vi "CAlex2_InitCuff.vi"(4 "ShankExtraWeight":dbl, 6 "ThighExtraWeight":dbl, 8 "error in (no error)":errorcluster, 10 "LegProperty":T1={"BodyDim(m)"={"ThighLt"=0.4, "ShankLt"=0.41, "HipWd"=0.32}, "BodyWt(kg)"={"Thigh"=0.0, "Shank"=0.0}, "CuffLoc(m)"={"HipCuffWd"=0.4, "HipCuffHt"=0.1, "HipCuffFwdShift"=0.0, "ThighCuffToKnee"=0.25, "ThighCuffDist"=0.0, "ShankCuffToKnee"=0.15}}, 11 "CAlex2 in":refnum<class "CAlex2.lvclass">) -> (0 "error out":errorcluster, 3 "CAlex2 out":refnum<class "CAlex2.lvclass">)   [LabVIEW 2015, in "CAlex2.lvclass"]
uses:
  CAlex2.lvclass
  TypeDef/LowerBodyDim.ctl
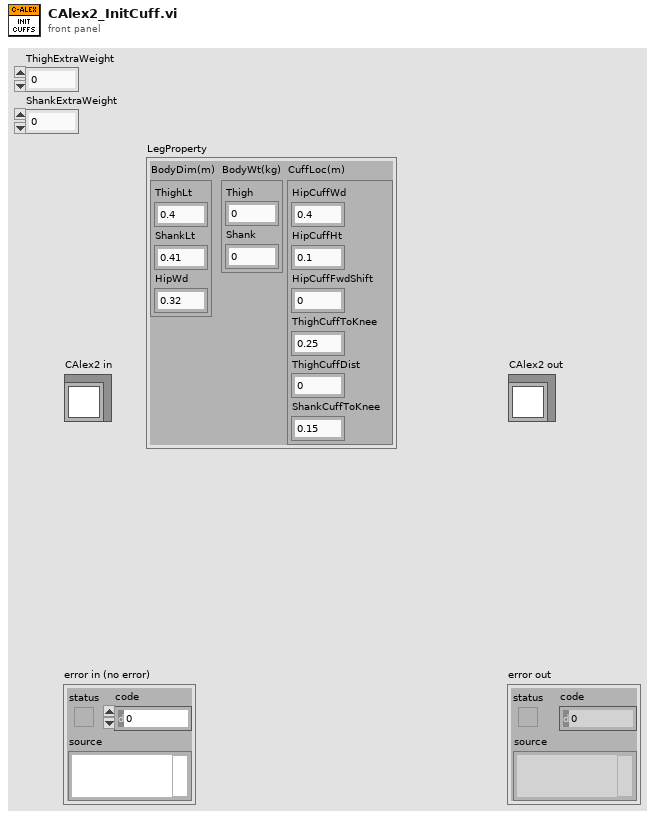
[diagram p1: front panel]
types:
  T1 = typedef "CAlex2.lvclass/LowerBodyDim.ctl" = cluster{"BodyDim(m)":cluster{"ThighLt":dbl, "ShankLt":dbl, "HipWd":dbl}, "BodyWt(kg)":cluster{"Thigh":dbl, "Shank":dbl}, "CuffLoc(m)":cluster{"HipCuffWd":dbl, "HipCuffHt":dbl, "HipCuffFwdShift":dbl, "ThighCuffToKnee":dbl, "ThighCuffDist":dbl, "ShankCuffToKnee":dbl}}
  T2 = enum16{"Thigh Cuff Low Lower Edge", "Thigh Cuff High Center"}
  T3 = typedef "CableSerialChain.lvclass/Cuff.ctl" = cluster{"BodyID":i32, "CoM(CuffCS)":T4, "Mass(kg)":dbl, "CablePts(CuffCS)":T4[], "Cuff->Body":T5}
  T4 = typedef "Bodies.lvclass/PointOnBody.ctl" = cluster{"Coord4":dbl[], "ID":i32}
  T5 = typedef "NI_Matrix.lvlib/RealMatrix.ctl" = dbl[][]
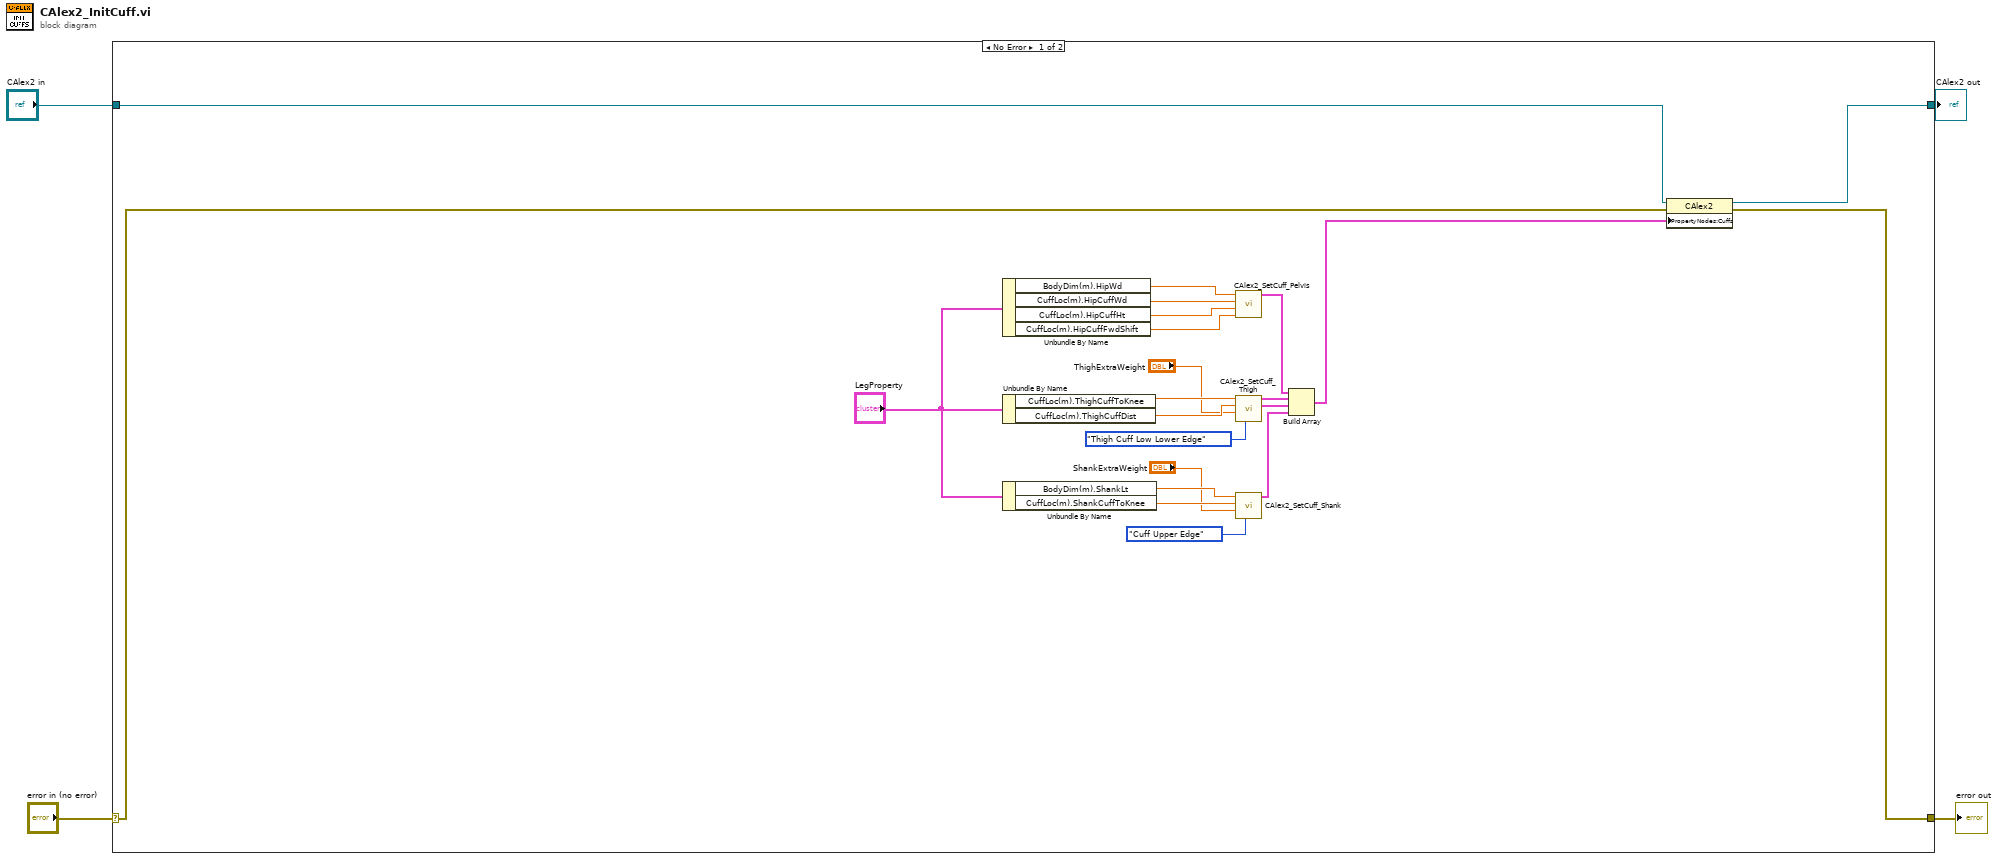
[diagram p0: block diagram]
diagram:
  n1 = case shown="No Error" "error in (no error)" {
    selector: "error in (no error)" -> [w7 w28]
    tunnel: [w24 w28] -> w3
    tunnel: [w25 w27] -> w1
    tunnel: "CAlex2 in" -> [w8 w27]
    frame No Error {
      n2 = Unbundle By Name("LegProperty") -> ("BodyDim(m).HipWd"=w15:dbl, "CuffLoc(m).HipCuffWd"=w13:dbl, "CuffLoc(m).HipCuffHt"=w14:dbl, "CuffLoc(m).HipCuffFwdShift"=w12:dbl)
      n3 = Unbundle By Name("LegProperty") -> ("CuffLoc(m).ThighCuffToKnee"=w11:dbl, "CuffLoc(m).ThighCuffDist"=w10:dbl)
      n4 = Unbundle By Name("LegProperty") -> ("BodyDim(m).ShankLt"=w19:dbl, "CuffLoc(m).ShankCuffToKnee"=w18:dbl)
      n5 = call "CAlex2_SetCuff_Pelvis.vi"("Hip Cuff Forward Shift"=w12, "Hip Cuff Height"=w14, "Hip Cuff Width"=w13, "Hip Width"=w15) -> ("Hip Cuff"=w23:T3)  [unwired: 7 in]
      n6 = call "CAlex2_SetCuff_Thigh.vi"("Knee Distance Reference"=T2."Thigh Cuff Low Lower Edge", "ExtraWeight"="ThighExtraWeight", "Thigh Cuff Low Distance From Bottom (Hole*0.00635)"=w10, "Knee Distance"=w11) -> ("Thigh Cuff Low"=w21:T3, "Thigh Cuff High"=w22:T3)  [unwired: 6 in]
      n7 = call "CAlex2_SetCuff_Shank.vi"("Reference Point"=enum16{"Cuff Center", "Cuff Upper Edge"}."Cuff Upper Edge", "ExtraWeight"="ShankExtraWeight", "Distance To Knee"=w18, "Shank Length"=w19) -> ("Shank Cuff"=w20:T3)  [unwired: 7 in]
      n8 = Build Array(w23, w22, w21, w20) -> (w26:T3[])
      n9 = property class="CAlex2"(reference=w8, error in=w7, "PropertyNodes:Cuffs"=w26) -> (reference out=w25:refnum<class "CAlex2.lvclass">, error out=w24:errorcluster)
    }
    frame Error {
    }
  }
  "error out" <- w3
  "CAlex2 out" <- w1
